vi "NI9219_DAQmx.vi"() -> ()   [LabVIEW 2022 SP3]
uses:
  <vilib>/DAQmx/read.llb/DAQmx Read (Analog 1D Wfm NChan NSamp).vi
  <vilib>/DAQmx/miscellaneous.llb/DAQmx Fill In Error Info.vi
panel:
  out "Waveform Chart 3":dynamicdata(graph)
  out "Waveform Chart 2":dynamicdata(graph)
  out "Waveform Chart":dynamicdata(graph)
  in  "Stop":bool
  in  "number of samples":i32=-1
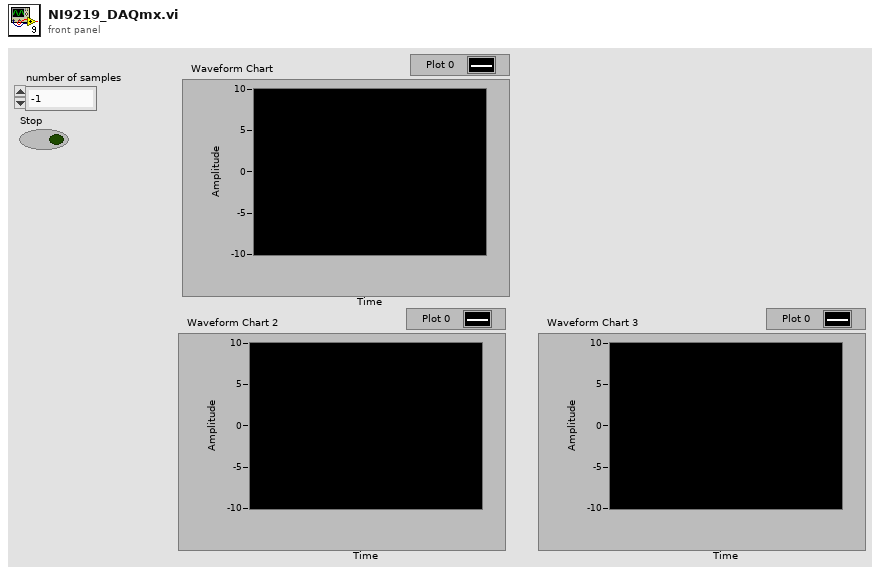
[diagram p1: front panel]
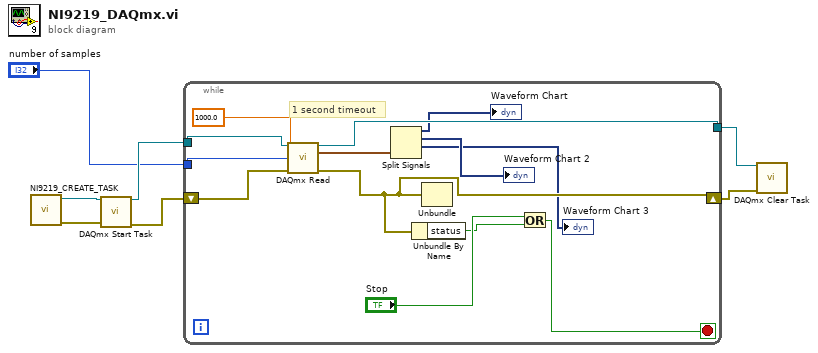
[diagram p0: block diagram]
diagram:
  n1 = call "NI9219_CREATE_TASK.vi"() -> ("error out"=w6:errorcluster, "task out"=w7:refnum<k21>)  [unwired: 10 in]
  n2 = call <vilib>:"DAQmx Start Task.vi"("task/channels in"=w7, "error in"=w6) -> ("task out"=w5:refnum<k21>, "error out"=w2:errorcluster)  [unwired: 12 in]
  n3 = while {
    tunnel: w5 -> [w20]
    tunnel: "number of samples" -> [w19]
    tunnel: [w16] -> w3
    shift-right: [w11] -> w1
    shift-left: w2 -> [w15]
    stop <- w12 stop-if-true
    # "1 second timeout"
    n4 = call-poly <vilib>:"DAQmx Read.vi"("task/channels in"=w20, "number of samples per channel"=w19, "timeout"=1000.0, "error in"=w15) -> ("task out"=w16:refnum<k21>, "data"=w17:waveform(dbl)[], "error out"=w11:errorcluster)  [unwired: 9 in]
    n5 = Split Signals(w17) -> (→"Waveform Chart":dynamicdata, →"Waveform Chart 2":dynamicdata, →"Waveform Chart 3":dynamicdata)  [unwired: 4 in, 1 out]
    n6 = Unbundle By Name(w11) -> ("status"=w13:bool)
    n7 = Unbundle(w11) -> ()  [unwired: 3 out]
    n8 = Or(x="Stop", y=w13) -> (x .or. y?=w12:bool)
  }
  n9 = call <vilib>:"DAQmx Clear Task.vi"("task in"=w3, "error in"=w1) -> ()  [unwired: 13 in, 1 out]
